vi "PicoScope2000aAdvancedTriggerSettings.vi"(0 "handle in":i16=16384, 2 "Auto Trigger (ms)":i32=1000, 3 "Trigger Conditions":T6 {"Condition Logic" items=["AND", "OR", "XOR"]}, 4 "Trigger Delay":u32, 5 "error in":errorcluster, 6 "Channel A Trigger Properties":T3={"thresholdUpper"=0, "thresholdUpperHysteresis"=0, "thresholdLower"=0, "thresholdLowerHysteresis"=0, "Threshold Mode"=0, "Direction"=0, "Available"=TRUE} {"Direction" items=["Above / Inside", "Below / Outside", "Rising / Enter", "Falling / Exit", "Rising or Falling / Enter or Exit", "Above Lower", "Below Lower", "Rising Lower", "Falling Lower", "Positive Runt", "Negative Runt"]; "Threshold Mode" items=["Level", "Window"]}, 7 "Channel D Trigger Properties":T3 {"Direction" items=["Above / Inside", "Below / Outside", "Rising / Enter", "Falling / Exit", "Rising or Falling / Enter or Exit", "Above Lower", "Below Lower", "Rising Lower", "Falling Lower", "Positive Runt", "Negative Runt"]; "Threshold Mode" items=["Level", "Window"]}, 8 "Channel B Trigger Properties":T3 {"Direction" items=["Above / Inside", "Below / Outside", "Rising / Enter", "Falling / Exit", "Rising or Falling / Enter or Exit", "Above Lower", "Below Lower", "Rising Lower", "Falling Lower", "Positive Runt", "Negative Runt"]; "Threshold Mode" items=["Level", "Window"]}, 10 "Digital Port  0":T2 {"Direction Channel 7" items=["Don't Care", "Low", "High", "Rising", "Falling"]; "Direction Channel 6" items=["Don't Care", "Low", "High", "Rising", "Falling"]; "Direction Channel 5" items=["Don't Care", "Low", "High", "Rising", "Falling"]; "Direction Channel 4" items=["Don't Care", "Low", "High", "Rising", "Falling"]; "Direction Channel 3" items=["Don't Care", "Low", "High", "Rising", "Falling"]; "Direction Channel 2" items=["Don't Care", "Low", "High", "Rising", "Falling"]; "Direction Channel 1" items=["Don't Care", "Low", "High", "Rising", "Falling"]; "Direction Channel 0" items=["Don't Care", "Low", "High", "Rising", "Falling"]}, 11 "Ext. Trigger Properties":T3 {"Direction" items=["Above / Inside", "Below / Outside", "Rising / Enter", "Falling / Exit", "Rising or Falling / Enter or Exit", "Above Lower", "Below Lower", "Rising Lower", "Falling Lower", "Positive Runt", "Negative Runt"]; "Threshold Mode" items=["Level", "Window"]}, 12 "Digital Port  1":T1 {"Direction Channel 15" items=["Don't Care", "Low", "High", "Rising", "Falling"]; "Direction Channel 14" items=["Don't Care", "Low", "High", "Rising", "Falling"]; "Direction Channel 13" items=["Don't Care", "Low", "High", "Rising", "Falling"]; "Direction Channel 12" items=["Don't Care", "Low", "High", "Rising", "Falling"]; "Direction Channel 11" items=["Don't Care", "Low", "High", "Rising", "Falling"]; "Direction Channel 10" items=["Don't Care", "Low", "High", "Rising", "Falling"]; "Direction Channel 9" items=["Don't Care", "Low", "High", "Rising", "Falling"]; "Direction Channel 8" items=["Don't Care", "Low", "High", "Rising", "Falling"]}, 13 "Aux. Trigger Properties":T3 {"Direction" items=["Above / Inside", "Below / Outside", "Rising / Enter", "Falling / Exit", "Rising or Falling / Enter or Exit", "Above Lower", "Below Lower", "Rising Lower", "Falling Lower", "Positive Runt", "Negative Runt"]; "Threshold Mode" items=["Level", "Window"]}, 16 "Channel C Trigger Properties":T3 {"Direction" items=["Above / Inside", "Below / Outside", "Rising / Enter", "Falling / Exit", "Rising or Falling / Enter or Exit", "Above Lower", "Below Lower", "Rising Lower", "Falling Lower", "Positive Runt", "Negative Runt"]; "Threshold Mode" items=["Level", "Window"]}, 17 "Pulse Width Qualifier Settings":T4={"Direction"=2, "Lower Limit"=0, "Upper Limit"=0, "Pulse Width Type"=0} {"Pulse Width Type" items=["None", "Less Than", "Greater Than", "In Range", "Out of Range"]; "Direction" items=["Rising"=2, "Falling"=3]}, 18 "Pulse Width Qualifier Conditions":T5 {"Condition Logic" items=["AND", "OR", "XOR"]}) -> (14 "handle out":i16=16384, 19 "error out":errorcluster)   [LabVIEW 2010]
doc: "This VI is an interface for the advanced trigger features of the oscilloscope (a simple trigger can be set using PicoScope3000aSettings.vi, in which case it is not necessary to use this VI)."
uses:
  ps2000a.dll
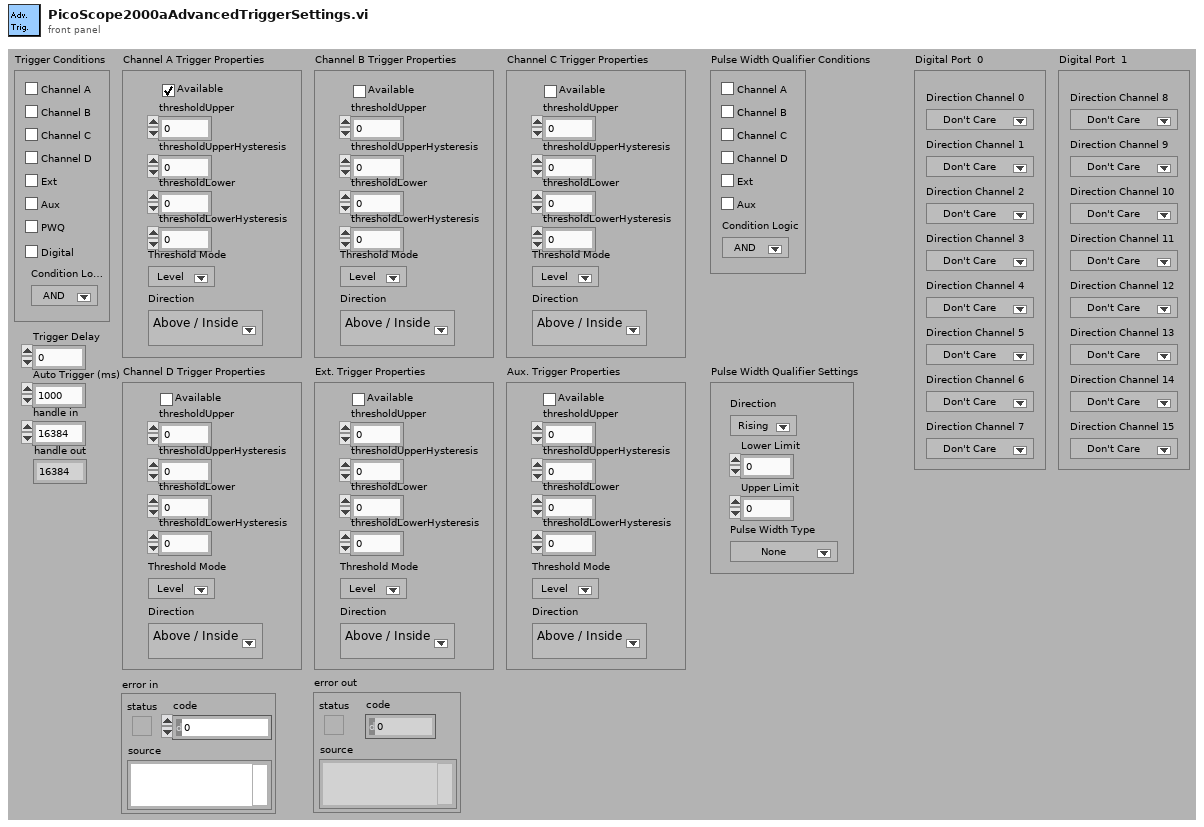
[diagram p1: front panel]
types:
  T1 = cluster{"Direction Channel 8":u16, "Direction Channel 9":u16, "Direction Channel 10":u16, "Direction Channel 11":u16, "Direction Channel 12":u16, "Direction Channel 13":u16, "Direction Channel 14":u16, "Direction Channel 15":u16}
  T2 = cluster{"Direction Channel 0":u16, "Direction Channel 1":u16, "Direction Channel 2":u16, "Direction Channel 3":u16, "Direction Channel 4":u16, "Direction Channel 5":u16, "Direction Channel 6":u16, "Direction Channel 7":u16}
  T3 = cluster{"thresholdUpper":i16, "thresholdUpperHysteresis":u16, "thresholdLower":i16, "thresholdLowerHysteresis":u16, "Threshold Mode":i32, "Direction":i32, "Available":bool}
  T4 = cluster{"Direction":i32, "Lower Limit":u32, "Upper Limit":u32, "Pulse Width Type":i32}
  T5 = cluster{"Channel A":bool, "Channel B":bool, "Channel C":bool, "Channel D":bool, "Aux":bool, "Condition Logic":u16, "Ext":bool}
  T6 = cluster{"Channel A":bool, "Channel B":bool, "Channel C":bool, "Channel D":bool, "Aux":bool, "PWQ":bool, "Condition Logic":u16, "Ext":bool, "Digital":bool}
  T7 = cluster{"thresholdUpper":i16, "thresholdUpperHysteresis":u16, "thresholdLower":i16, "thresholdLowerHysteresis":u16, "Threshold Mode":i32, "Direction":i32, "Available":bool}[]
  T8 = cluster{"[0]":i32, "[1]":i32, "[2]":i32, "[3]":i32, "[4]":i32, "[5]":i32, "[6]":i32, "[7]":i32, "[8]":i32}
  T9 = cluster{"status":bool, "code":u32, "source":string}
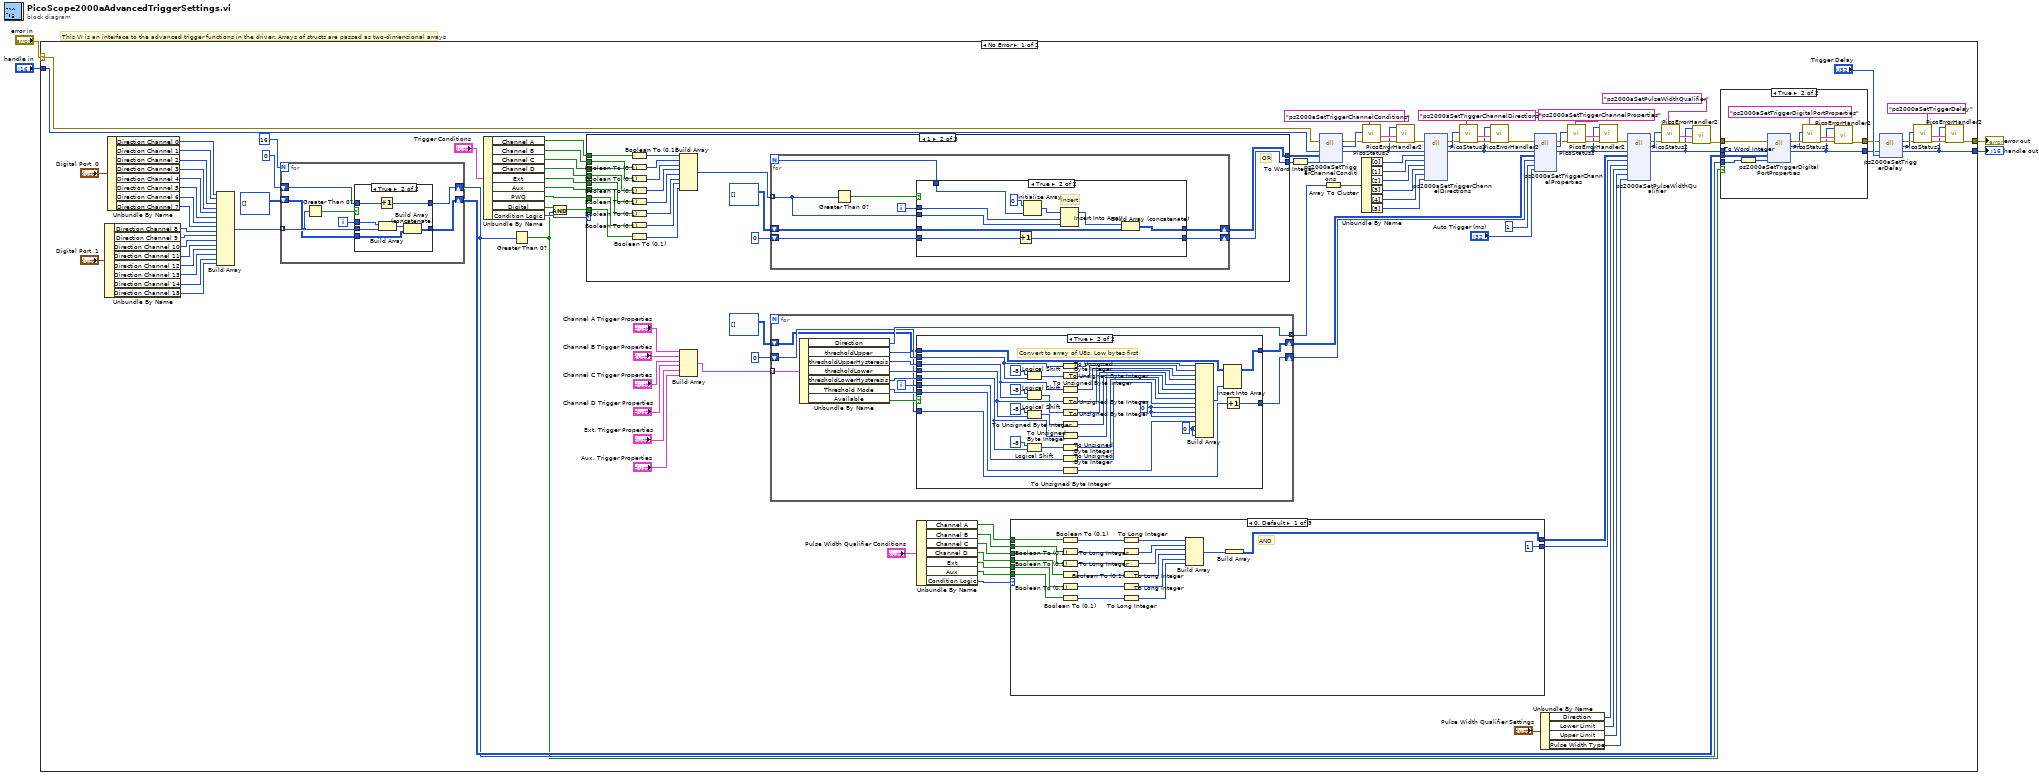
[diagram p0: block diagram]
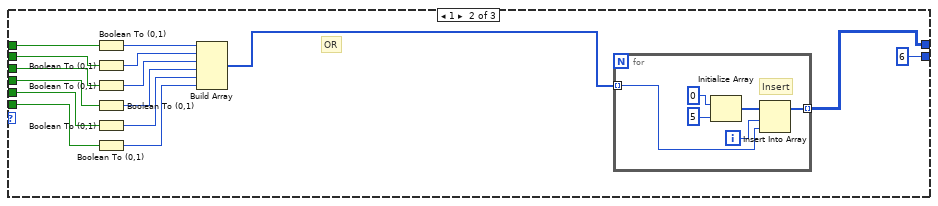
[diagram p4: hidden frame]
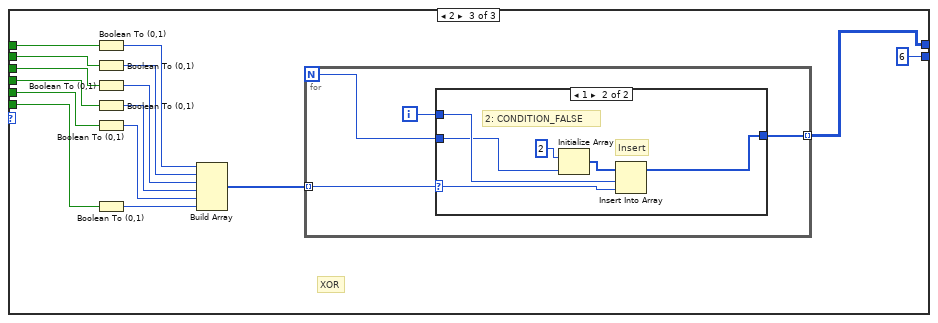
[diagram p5: hidden frame]
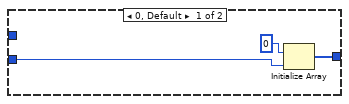
[diagram p6: hidden frame]
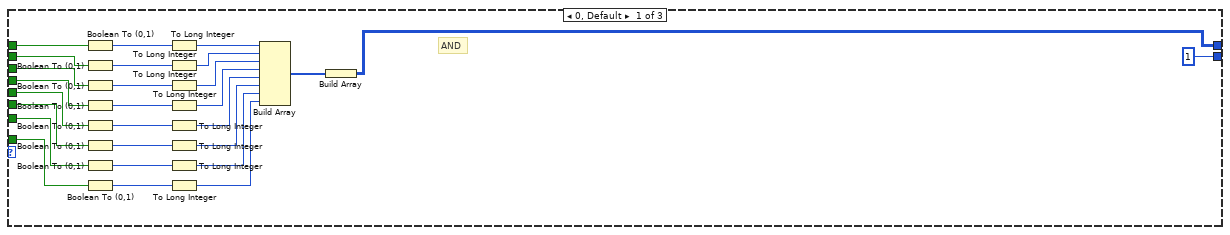
[diagram p8: hidden frame]
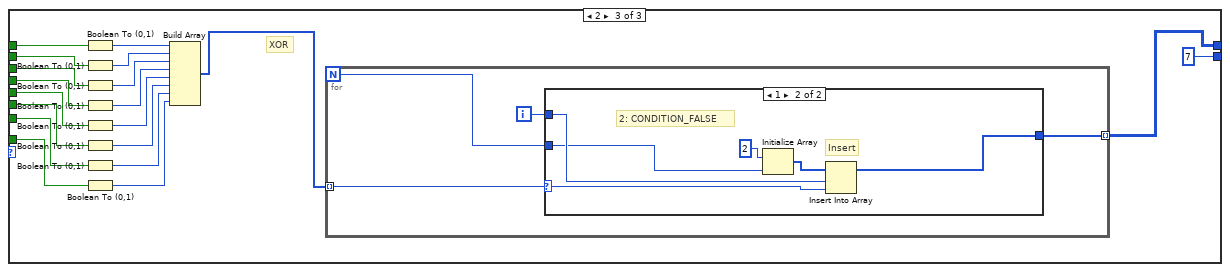
[diagram p10: hidden frame]
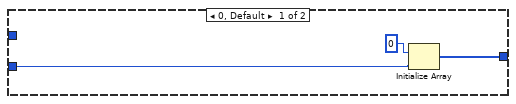
[diagram p11: hidden frame]
diagram:
  # "This VI is an interface to the advanced trigger functions in the driver. Arrays of structs are passed as two-dimensional arrays"
  n1 = case shown="No Error" "error in" {
    selector: "error in" -> [w81 w366]
    tunnel: "handle in" -> [w85 w367]
    tunnel: [w5 w367] -> w2
    tunnel: [w71 w366] -> w1
    frame No Error {
      n2 = Unbundle By Name("Digital Port  1") -> ("Direction Channel 8"=w41:u16, "Direction Channel 9"=w40:u16, "Direction Channel 10"=w39:u16, "Direction Channel 11"=w38:u16, "Direction Channel 12"=w37:u16, "Direction Channel 13"=w36:u16, "Direction Channel 14"=w35:u16, "Direction Channel 15"=w34:u16)
      n3 = Unbundle By Name("Digital Port  0") -> ("Direction Channel 0"=w54:u16, "Direction Channel 1"=w53:u16, "Direction Channel 2"=w52:u16, "Direction Channel 3"=w51:u16, "Direction Channel 4"=w50:u16, "Direction Channel 5"=w49:u16, "Direction Channel 6"=w48:u16, "Direction Channel 7"=w47:u16)
      n4 = Build Array(w54, w53, w52, w51, w50, w49, w48, w47, w41, w40, w39, w38, w37, w36, w35, w34) -> (w44:u16[])
      n5 = for {
        N: 16 -> [_]
        tunnel: w44 -> [w138] mode=indexing
        shift-right: [w137] -> w29
        shift-left: i32[][] [] -> [w136]
        shift-right: [w135] -> w26
        shift-left: 0 -> [w134]
        i -> [w139]
        n6 = Greater Than 0?(x=w138) -> (x > 0?=w140:bool)
        n7 = case shown="True" w140 {
          tunnel: w139 -> [_ w149]
          tunnel: w138 -> [_ w148]
          tunnel: [w142 w146] -> w137
          tunnel: w136 -> [w142 w145]
          tunnel: [w141 w144] -> w135
          tunnel: w134 -> [w141 w143]
          frame False {
          }
          frame True {
            n8 = Increment(x=w143) -> (x+1=w144:i32)
            n9 = Build Array(w149, w148) -> (w147:i32[])
            n10 = Build Array (concatenate)(w147, w145) -> (w146:i32[][])
          }
        }
      }
      n11 = Unbundle By Name("Trigger Conditions") -> ("Channel A"=w61:bool, "Channel B"=w60:bool, "Channel C"=w59:bool, "Channel D"=w58:bool, "Ext"=w57:bool, "Aux"=w56:bool, "PWQ"=w55:bool, "Digital"=w28:bool, "Condition Logic"=w62:u16)
      n12 = Greater Than 0?(x=w26) -> (x > 0?=w25:bool)
      n13 = And(x=w28, y=w25) -> (x .and. y?=w27:bool)
      n14 = case shown="1" w62 {
        tunnel: [w277 w305 w344] -> w117
        tunnel: [i16 1 w303 i16 7] -> w24
        tunnel: w61 -> [w273 w300 w341]
        tunnel: w60 -> [w272 w299 w340]
        tunnel: w59 -> [w271 w298 w339]
        tunnel: w58 -> [w270 w297 w338]
        tunnel: w57 -> [w269 w296 w337]
        tunnel: w56 -> [w268 w295 w336]
        tunnel: w55 -> [w267 w294 w335]
        tunnel: w27 -> [w266 w293 w334]
        frame 0, Default {
          # "AND"
          n15 = Boolean To (0,1)(Boolean=w273) -> (0, 1=w292:i16)
          n16 = Boolean To (0,1)(Boolean=w272) -> (0, 1=w291:i16)
          n17 = Boolean To (0,1)(Boolean=w271) -> (0, 1=w290:i16)
          n18 = Boolean To (0,1)(Boolean=w270) -> (0, 1=w289:i16)
          n19 = Boolean To (0,1)(Boolean=w269) -> (0, 1=w288:i16)
          n20 = Boolean To (0,1)(Boolean=w268) -> (0, 1=w287:i16)
          n21 = Boolean To (0,1)(Boolean=w267) -> (0, 1=w286:i16)
          n22 = Boolean To (0,1)(Boolean=w266) -> (0, 1=w275:i16)
          n23 = To Long Integer(number=w292) -> (32bit integer=w285:i32)
          n24 = To Long Integer(number=w291) -> (32bit integer=w284:i32)
          n25 = To Long Integer(number=w290) -> (32bit integer=w283:i32)
          n26 = To Long Integer(number=w289) -> (32bit integer=w282:i32)
          n27 = To Long Integer(number=w288) -> (32bit integer=w281:i32)
          n28 = To Long Integer(number=w287) -> (32bit integer=w280:i32)
          n29 = To Long Integer(number=w286) -> (32bit integer=w279:i32)
          n30 = To Long Integer(number=w275) -> (32bit integer=w274:i32)
          n31 = Build Array(w285, w284, w283, w282, w281, w280, w279, w274) -> (w278:i32[])
          n32 = Build Array(w278) -> (w277:i32[][])
        }
        frame 1 {
          # "OR"
          n33 = Boolean To (0,1)(Boolean=w300) -> (0, 1=w307:i16)
          n34 = Boolean To (0,1)(Boolean=w299) -> (0, 1=w308:i16)
          n35 = Boolean To (0,1)(Boolean=w298) -> (0, 1=w309:i16)
          n36 = Boolean To (0,1)(Boolean=w297) -> (0, 1=w310:i16)
          n37 = Boolean To (0,1)(Boolean=w296) -> (0, 1=w311:i16)
          n38 = Boolean To (0,1)(Boolean=w295) -> (0, 1=w312:i16)
          n39 = Boolean To (0,1)(Boolean=w294) -> (0, 1=w313:i16)
          n40 = Boolean To (0,1)(Boolean=w293) -> (0, 1=w301:i16)
          n41 = Build Array(w307, w308, w309, w310, w311, w312, w313, w301) -> (w306:i16[])
          n42 = for {
            N -> [w314]
            tunnel: w306 -> [w318] mode=indexing
            shift-right: [w317] -> w305
            shift-left: i32[][] [] -> [w321]
            shift-right: [w315] -> w303
            shift-left: 0 -> [w316]
            i -> [w320]
            n43 = Greater Than 0?(x=w318) -> (x > 0?=w319:bool)
            n44 = case shown="True" w319 {
              tunnel: w321 -> [w323 w327]
              tunnel: w320 -> [_ w331]
              tunnel: w318 -> [_ w330]
              tunnel: [w323 w329] -> w317
              tunnel: w316 -> [w322 w326]
              tunnel: [w322 w325] -> w315
              tunnel: w314 -> [_ w324]
              frame False {
              }
              frame True {
                # "Insert"
                n45 = Increment(x=w326) -> (x+1=w325:i32)
                n46 = Initialize Array(0 ("element"), w324) -> (w332:i32[])
                n47 = Insert Into Array(array=w332, index=w331, new element=w330) -> (w328:i32[])
                n48 = Build Array (concatenate)(w328, w327) -> (w329:i32[][])
              }
            }
          }
        }
        frame 2 {
          # "XOR"
          n49 = Boolean To (0,1)(Boolean=w341) -> (0, 1=w346:i16)
          n50 = Boolean To (0,1)(Boolean=w340) -> (0, 1=w347:i16)
          n51 = Boolean To (0,1)(Boolean=w339) -> (0, 1=w348:i16)
          n52 = Boolean To (0,1)(Boolean=w338) -> (0, 1=w349:i16)
          n53 = Boolean To (0,1)(Boolean=w337) -> (0, 1=w350:i16)
          n54 = Boolean To (0,1)(Boolean=w336) -> (0, 1=w351:i16)
          n55 = Boolean To (0,1)(Boolean=w335) -> (0, 1=w352:i16)
          n56 = Boolean To (0,1)(Boolean=w334) -> (0, 1=w342:i16)
          n57 = Build Array(w346, w347, w348, w349, w350, w351, w352, w342) -> (w345:i16[])
          n58 = for {
            N -> [w353]
            tunnel: w345 -> [w354] mode=indexing
            tunnel: [w356] -> w344 mode=indexing
            i -> [w355]
            n59 = case shown="1" w354 {
              selector: w354 -> [_ w362]
              tunnel: [w358 w363] -> w356
              tunnel: w355 -> [_ w361]
              tunnel: w353 -> [w357 w360]
              frame 0, Default {
                n60 = Initialize Array(0 ("element"), w357) -> (w358:i32[])
              }
              frame 1 {
                # "2: CONDITION_FALSE"
                # "Insert"
                n61 = Initialize Array(2 ("element"), w360) -> (w364:i32[])
                n62 = Insert Into Array(array=w364, index=w361, new element=w362) -> (w363:i32[])
              }
            }
          }
        }
      }
      n63 = Build Array("Channel A Trigger Properties", "Channel B Trigger Properties", "Channel C Trigger Properties", "Channel D Trigger Properties", "Ext. Trigger Properties", "Aux. Trigger Properties") -> (w115:T7)
      n64 = for {
        tunnel: w115 -> [w227] mode=indexing
        tunnel: [w226] -> w114 mode=indexing
        shift-right: [w223] -> w65
        shift-left: i16 0 -> [w222]
        shift-right: [w220] -> w63
        shift-left: u8[][] [] -> [w221]
        i -> [w224]
        n65 = Unbundle By Name(w227) -> ("Direction"=w226:i32, "thresholdUpper"=w232:i16, "thresholdUpperHysteresis"=w231:u16, "thresholdLower"=w230:i16, "thresholdLowerHysteresis"=w229:u16, "Threshold Mode"=w228:i32, "Available"=w225:bool)
        n66 = case shown="True" w225 {
          tunnel: w232 -> [_ w264]
          tunnel: w231 -> [_ w256]
          tunnel: w230 -> [_ w255]
          tunnel: w229 -> [_ w254]
          tunnel: w228 -> [_ w245]
          tunnel: w224 -> [_ w240]
          tunnel: [w234 w239] -> w223
          tunnel: w222 -> [w234 w238]
          tunnel: [w233 w236] -> w220
          tunnel: w221 -> [w233 w235]
          frame False {
          }
          frame True {
            w243 = u8 0 ("element")
            w244 = u8 0 ("element")
            # "Convert to array of U8s, Low bytes first"
            n67 = Logical Shift(y=i16 -8, x=w264) -> (x << y=w263:i16)
            n68 = Logical Shift(y=i16 -8, x=w256) -> (x << y=w262:u16)
            n69 = Logical Shift(y=i16 -8, x=w255) -> (x << y=w259:i16)
            n70 = Logical Shift(y=i16 -8, x=w254) -> (x << y=w258:u16)
            n71 = To Unsigned Byte Integer(number=w264) -> (unsigned 8bit integer=w253:u8)
            n72 = To Unsigned Byte Integer(number=w263) -> (unsigned 8bit integer=w252:u8)
            n73 = To Unsigned Byte Integer(number=w256) -> (unsigned 8bit integer=w251:u8)
            n74 = To Unsigned Byte Integer(number=w262) -> (unsigned 8bit integer=w250:u8)
            n75 = To Unsigned Byte Integer(number=w255) -> (unsigned 8bit integer=w249:u8)
            n76 = To Unsigned Byte Integer(number=w259) -> (unsigned 8bit integer=w248:u8)
            n77 = To Unsigned Byte Integer(number=w254) -> (unsigned 8bit integer=w247:u8)
            n78 = To Unsigned Byte Integer(number=w258) -> (unsigned 8bit integer=w246:u8)
            n79 = To Unsigned Byte Integer(number=w240) -> (unsigned 8bit integer=w241:u8)
            n80 = To Unsigned Byte Integer(number=w245) -> (unsigned 8bit integer=w242:u8)
            n81 = Build Array(w253, w252, w251, w250, w249, w248, w247, w246, w241, w244, w244, w244, w242, w243, w243, w243) -> (w237:u8[])
            n82 = Insert Into Array(array=w235, new element=w237) -> (w236:u8[][])  [unwired: 2 in]
            n83 = Increment(x=w238) -> (x+1=w239:i16)
          }
        }
      }
      n84 = Unbundle By Name("Pulse Width Qualifier Conditions") -> ("Channel A"=w104:bool, "Channel B"=w103:bool, "Channel C"=w102:bool, "Channel D"=w101:bool, "Ext"=w100:bool, "Aux"=w91:bool, "Condition Logic"=w92:u16)
      n85 = case shown="0, Default" w92 {
        tunnel: w104 -> [w170 w185 w206]
        tunnel: w103 -> [w164 w184 w205]
        tunnel: w102 -> [w163 w183 w204]
        tunnel: w101 -> [w162 w182 w203]
        tunnel: w100 -> [w161 w173 w194]
        tunnel: [w154 w175 w196] -> w99
        tunnel: [i16 1 i16 6 i16 6] -> w98
        tunnel: w91 -> [w151 w172 w193]
        frame 0, Default {
          # "AND"
          n86 = Boolean To (0,1)(Boolean=w170) -> (0, 1=w169:i16)
          n87 = Boolean To (0,1)(Boolean=w164) -> (0, 1=w168:i16)
          n88 = Boolean To (0,1)(Boolean=w163) -> (0, 1=w167:i16)
          n89 = Boolean To (0,1)(Boolean=w162) -> (0, 1=w166:i16)
          n90 = Boolean To (0,1)(Boolean=w161) -> (0, 1=w165:i16)
          n91 = Boolean To (0,1)(Boolean=w151) -> (0, 1=w152:i16)
          n92 = To Long Integer(number=w169) -> (32bit integer=w160:i32)
          n93 = To Long Integer(number=w168) -> (32bit integer=w159:i32)
          n94 = To Long Integer(number=w167) -> (32bit integer=w158:i32)
          n95 = To Long Integer(number=w166) -> (32bit integer=w157:i32)
          n96 = To Long Integer(number=w165) -> (32bit integer=w156:i32)
          n97 = To Long Integer(number=w152) -> (32bit integer=w150:i32)
          n98 = Build Array(w160, w159, w158, w157, w156, w150) -> (w155:i32[])
          n99 = Build Array(w155) -> (w154:i32[][])
        }
        frame 1 {
          # "OR"
          n100 = Boolean To (0,1)(Boolean=w185) -> (0, 1=w177:i16)
          n101 = Boolean To (0,1)(Boolean=w184) -> (0, 1=w178:i16)
          n102 = Boolean To (0,1)(Boolean=w183) -> (0, 1=w179:i16)
          n103 = Boolean To (0,1)(Boolean=w182) -> (0, 1=w180:i16)
          n104 = Boolean To (0,1)(Boolean=w173) -> (0, 1=w181:i16)
          n105 = Boolean To (0,1)(Boolean=w172) -> (0, 1=w171:i16)
          n106 = Build Array(w177, w178, w179, w180, w181, w171) -> (w176:i16[])
          n107 = for {
            tunnel: w176 -> [w187] mode=indexing
            tunnel: [w186] -> w175 mode=indexing
            i -> [w188]
            # "Insert"
            n108 = Initialize Array(0 ("element"), 5 ("dimension size")) -> (w189:i32[])
            n109 = Insert Into Array(array=w189, index=w188, new element=w187) -> (w186:i32[])
          }
        }
        frame 2 {
          # "XOR"
          n110 = Boolean To (0,1)(Boolean=w206) -> (0, 1=w198:i16)
          n111 = Boolean To (0,1)(Boolean=w205) -> (0, 1=w199:i16)
          n112 = Boolean To (0,1)(Boolean=w204) -> (0, 1=w200:i16)
          n113 = Boolean To (0,1)(Boolean=w203) -> (0, 1=w201:i16)
          n114 = Boolean To (0,1)(Boolean=w194) -> (0, 1=w202:i16)
          n115 = Boolean To (0,1)(Boolean=w193) -> (0, 1=w192:i16)
          n116 = Build Array(w198, w199, w200, w201, w202, w192) -> (w197:i16[])
          n117 = for {
            N -> [w207]
            tunnel: w197 -> [w210] mode=indexing
            tunnel: [w208] -> w196 mode=indexing
            i -> [w209]
            n118 = case shown="1" w210 {
              selector: w210 -> [_ w216]
              tunnel: [w212 w217] -> w208
              tunnel: w209 -> [_ w215]
              tunnel: w207 -> [w211 w214]
              frame 0, Default {
                n119 = Initialize Array(0 ("element"), w211) -> (w212:i32[])
              }
              frame 1 {
                # "2: CONDITION_FALSE"
                # "Insert"
                n120 = Initialize Array(2 ("element"), w214) -> (w218:i32[])
                n121 = Insert Into Array(array=w218, index=w215, new element=w216) -> (w217:i32[])
              }
            }
          }
        }
      }
      n122 = To Word Integer(number=w24) -> (16bit integer=w23:i16)
      n123 = dll-call lib="ps2000a.dll" fn="ps2000aSetTriggerChannelConditions" ("ps3000.dll:_ps3000_open_unit@0")(error in=w81, "handle"=w85, "conditions"=w117, "nConditions"=w23) -> (error out=w83:errorcluster, "PICO_STATUS"=w84:u32, "handle"=w19:i16)  [unwired: 4 in, 1 out]
      n124 = Array To Cluster(array=w114) -> (cluster=w113:T8)
      n125 = Unbundle By Name(w113) -> ("[0]"=w112:i32, "[1]"=w111:i32, "[2]"=w110:i32, "[3]"=w109:i32, "[4]"=w108:i32, "[5]"=w107:i32)
      n126 = call "PicoStatus2.vi"("PICO source"="ps2000aSetTriggerChannelConditions" ("source"), "Error in"=w83, "PICO STATUS"=w84) -> ("error out"=w22:errorcluster, "PICO_STATUS out"=w21:T9)  [unwired: 5 in]
      n127 = call "PicoErrorHandler2.vi"("error in (no error)"=w22, "PICO_STATUS in"=w21, "handle In"=w19) -> ("error out"=w20:errorcluster)  [unwired: 8 in]
      n128 = dll-call lib="ps2000a.dll" fn="ps2000aSetTriggerChannelDirections" ("ps3000.dll:_ps3000_open_unit@0")(error in=w20, "handle"=w19, "channelA"=w112, "channelB"=w111, "channelC"=w110, "channelD"=w109, "ext"=w108, "aux"=w107) -> (error out=w79:errorcluster, "PICO_STATUS"=w80:u32, "handle"=w16:i16)  [unwired: 8 in, 1 out]
      n129 = call "PicoStatus2.vi"("PICO source"="ps2000aSetTriggerChannelDirections" ("source"), "Error in"=w79, "PICO STATUS"=w80) -> ("error out"=w18:errorcluster, "PICO_STATUS out"=w17:T9)  [unwired: 5 in]
      n130 = call "PicoErrorHandler2.vi"("error in (no error)"=w18, "PICO_STATUS in"=w17, "handle In"=w16) -> ("error out"=w15:errorcluster)  [unwired: 8 in]
      n131 = dll-call lib="ps2000a.dll" fn="ps2000aSetTriggerChannelProperties" ("ps3000.dll:_ps3000_open_unit@0")(error in=w15, "handle"=w16, "channelProperties"=w63, "nChannelProperties"=w65, "auxOutputEnable"=i16 1, "autoTriggerMilliseconds"="Auto Trigger (ms)") -> (error out=w77:errorcluster, "PICO_STATUS"=w78:u32, "handle"=w12:i16)  [unwired: 6 in, 1 out]
      n132 = Unbundle By Name("Pulse Width Qualifier Settings") -> ("Direction"=w96:i32, "Lower Limit"=w95:u32, "Upper Limit"=w94:u32, "Pulse Width Type"=w93:i32)
      n133 = call "PicoStatus2.vi"("PICO source"="ps2000aSetTriggerChannelProperties" ("source"), "Error in"=w77, "PICO STATUS"=w78) -> ("error out"=w14:errorcluster, "PICO_STATUS out"=w13:T9)  [unwired: 5 in]
      n134 = call "PicoErrorHandler2.vi"("error in (no error)"=w14, "PICO_STATUS in"=w13, "handle In"=w12) -> ("error out"=w11:errorcluster)  [unwired: 8 in]
      n135 = dll-call lib="ps2000a.dll" fn="ps2000aSetPulseWidthQualifier" ("ps3000.dll:_ps3000_open_unit@0")(error in=w11, "handle"=w12, "conditions"=w99, "nConditions"=w98, "direction"=w96, "lower"=w95, "upper"=w94, "type"=w93) -> (error out=w75:errorcluster, "PICO_STATUS"=w76:u32, "handle"=w8:i16)  [unwired: 8 in, 1 out]
      n136 = call "PicoStatus2.vi"("PICO source"="ps2000aSetPulseWidthQualifier" ("source"), "Error in"=w75, "PICO STATUS"=w76) -> ("error out"=w10:errorcluster, "PICO_STATUS out"=w9:T9)  [unwired: 5 in]
      n137 = call "PicoErrorHandler2.vi"("error in (no error)"=w10, "PICO_STATUS in"=w9, "handle In"=w8) -> ("error out"=w7:errorcluster)  [unwired: 8 in]
      n138 = case shown="True" w25 {
        tunnel: w7 -> [w121 w132]
        tunnel: w8 -> [w120 w131]
        tunnel: [w121 w123] -> w31
        tunnel: [w120 w122] -> w30
        tunnel: w26 -> [_ w126]
        tunnel: w29 -> [_ w128]
        frame False {
        }
        frame True {
          n139 = To Word Integer(number=w126) -> (16bit integer=w127:i16)
          n140 = dll-call lib="ps2000a.dll" fn="ps2000aSetTriggerDigitalPortProperties"(error in=w132, "handle"=w131, "digitalDirections"=w128, "nDigitalDirections"=w127) -> (error out=w130:errorcluster, "PICO_STATUS"=w129:u32, "handle"=w122:i16)  [unwired: 4 in, 1 out]
          n141 = call "PicoStatus2.vi"("PICO source"="ps2000aSetTriggerDigitalPortProperties" ("source"), "Error in"=w130, "PICO STATUS"=w129) -> ("error out"=w125:errorcluster, "PICO_STATUS out"=w124:T9)  [unwired: 5 in]
          n142 = call "PicoErrorHandler2.vi"("error in (no error)"=w125, "PICO_STATUS in"=w124, "handle In"=w122) -> ("error out"=w123:errorcluster)  [unwired: 8 in]
        }
      }
      n143 = dll-call lib="ps2000a.dll" fn="ps2000aSetTriggerDelay" ("ps3000.dll:_ps3000_open_unit@0")(error in=w31, "handle"=w30, "delay"="Trigger Delay") -> (error out=w73:errorcluster, "PICO_STATUS"=w74:u32, "handle"=w5:i16)  [unwired: 3 in, 1 out]
      n144 = call "PicoStatus2.vi"("PICO source"="ps2000aSetTriggerDelay" ("source"), "Error in"=w73, "PICO STATUS"=w74) -> ("error out"=w72:errorcluster, "PICO_STATUS out"=w6:T9)  [unwired: 5 in]
      n145 = call "PicoErrorHandler2.vi"("error in (no error)"=w72, "PICO_STATUS in"=w6, "handle In"=w5) -> ("error out"=w71:errorcluster)  [unwired: 8 in]
    }
    frame Error {
    }
  }
  "handle out" <- w2
  "error out" <- w1
